vi "ALTS-2015 Three Button Error Dialog.vi"(8 "Error In":errorcluster, 11 "Window Title":string="Error in Analogue Channel") -> (0 "Error Out":errorcluster, 3 "Which Button?":T1(ring)=enum."Center Button")   [LabVIEW 2013]
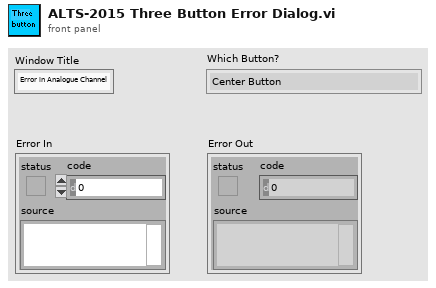
[diagram p1: front panel]
types:
  T1 = enum16{"Left Button", "Center Button", "Right Button", "Window Close"}
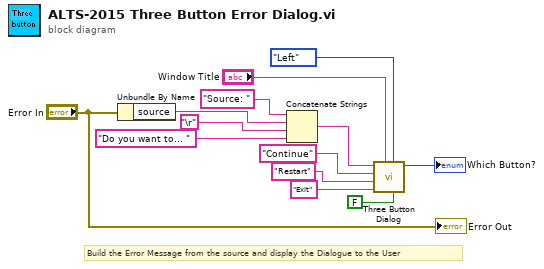
[diagram p0: block diagram]
diagram:
  # "Build the Error Message from the source and display the Dialogue to the User"
  n1 = Unbundle By Name("Error In") -> ("source"=w13:string)
  n2 = Concatenate Strings("Source: " ("Left Button Text (Yes)"), w13, "\r", "Do you want to... " ("string")) -> (w9:string)
  n3 = call <vilib>:"Three Button Dialog.vi"("Allow user to close window? (TRUE)"=FALSE, "Justify Message (Left)"=enum16{"Left", "Center", "Right"}."Left", "Window Title (\"\")"="Window Title", "Right Button Text (\"Cancel\")"="Exit" ("Right Button Text(Cancel)"), "Center Button Text (\"No\")"="Restart" ("Center Button Text(No)"), "Left Button Text (\"Yes\")"="Continue" ("Left Button Text (Yes)"), "message"=w9) -> ("Which Button?"=→"Which Button?":T1)  [unwired: 4 in]
  "Error Out" <- "Error In"
